vi "initialise.vi"(8 "error in (no error)":errorcluster, 11 "SpinCore in":refnum<class "SpinCore.lvclass">) -> (0 "error out":errorcluster, 3 "SpinCore out":refnum<class "SpinCore.lvclass">)   [LabVIEW 2009, in "Hardware.lvlib" / "Channels.lvlib" / "SpinCore.lvclass"]
doc: "Sets the Board number and clock rate."
uses:
  SpinCore.lvclass
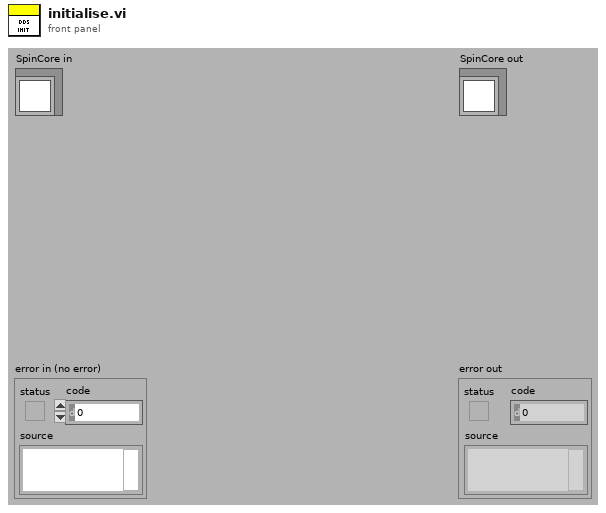
[diagram p1: front panel]
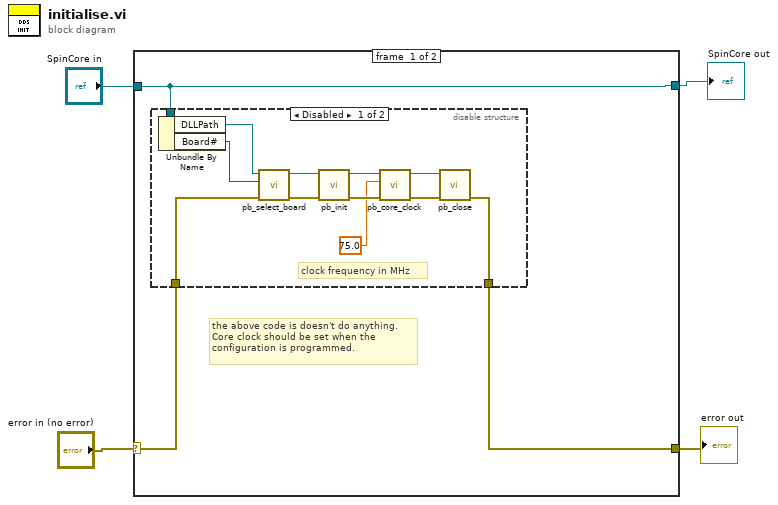
[diagram p0: block diagram]
diagram:
  n1 = case shown="No Error" "error in (no error)" {
    selector: "error in (no error)" -> [w7 w22]
    tunnel: [w5 w21] -> w3
    tunnel: "SpinCore in" -> [w5 w21]
    tunnel: [w6 w22] -> w1
    frame #0 {
      # "the above code is doesn't do anything.\nCore clock should be set when the \nconfiguration is programmed."
      n2 = disable-structure shown="Disabled" {
        disable-tunnel: w7 -> [w13 w20]
        disable-tunnel: [w12 w20] -> w6
        disable-tunnel: w5 -> [w8 _]
        frame #0 {
          # "clock frequency in MHz"
          n3 = Unbundle By Name(w8) -> ("DLLPath"=w10:path, "Board#"=w9:i32)
          n4 = call <userlib>:"pb_select_board.vi"("error in (no error)"=w13, "board_num"=w9, "path in"=w10) -> ("error out"=w19:errorcluster, "path out"=w18:path)  [unwired: 7 in]
          n5 = call <userlib>:"pb_init.vi"("error in (no error)"=w19, "path in"=w18) -> ("error out"=w17:errorcluster, "path out"=w16:path)  [unwired: 8 in]
          n6 = call <userlib>:"pb_core_clock.vi"("error in (no error)"=w17, "clock_freq (MHz)"=75.0, "path in"=w16) -> ("error out"=w15:errorcluster, "path out"=w14:path)  [unwired: 7 in]
          n7 = call <userlib>:"pb_close.vi"("error in (no error)"=w15, "path in"=w14) -> ("error out"=w12:errorcluster)  [unwired: 8 in, 1 out]
        }
        frame #1 {
        }
      }
    }
    frame #1 {
    }
  }
  "error out" <- w1
  "SpinCore out" <- w3
